vi "Header Size.vi"() -> (3 "Header Size":i32=9)   [LabVIEW 2020]
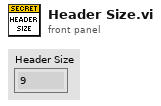
[diagram p1: front panel]
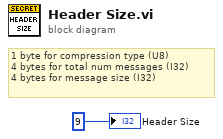
[diagram p0: block diagram]
diagram:
  # "1 byte for compression type (U8)\n4 bytes for total num messages (I32)\n4 bytes for message size (I32)"
  "Header Size" <- 9
